vi "VSG_SET-GET_AMPL_1.00.vi"(4 "delay after set (s)":dbl caption="Delay Time (s)", 6 "Get Power Only (T)":bool, 7 "Offset":dbl, 8 "error in":errorcluster {"code" format="%.0x"}, 9 "Set Power (num)":dbl=-25.0, 10 "Set Power(str)":string, 11 "Session In":refnum<visa-resource-name>="GPIB0::18::INSTR") -> (0 "error out":errorcluster {"code" format="%.0x"}, 1 "Get Power":dbl=-25.0, 2 "Get Power (str)":string="-25.000", 3 "Session Out":refnum<visa-resource-name>="GPIB0::18::INSTR")   [LabVIEW 2018]
doc: "Set/Get the ESG RF Amplitude in current units."
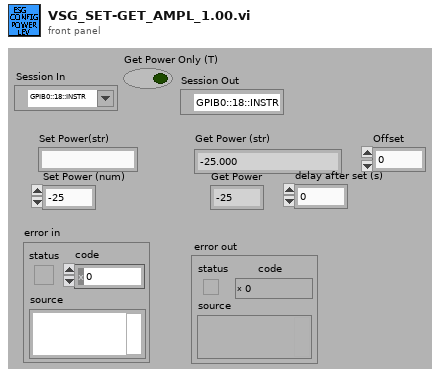
[diagram p1: front panel]
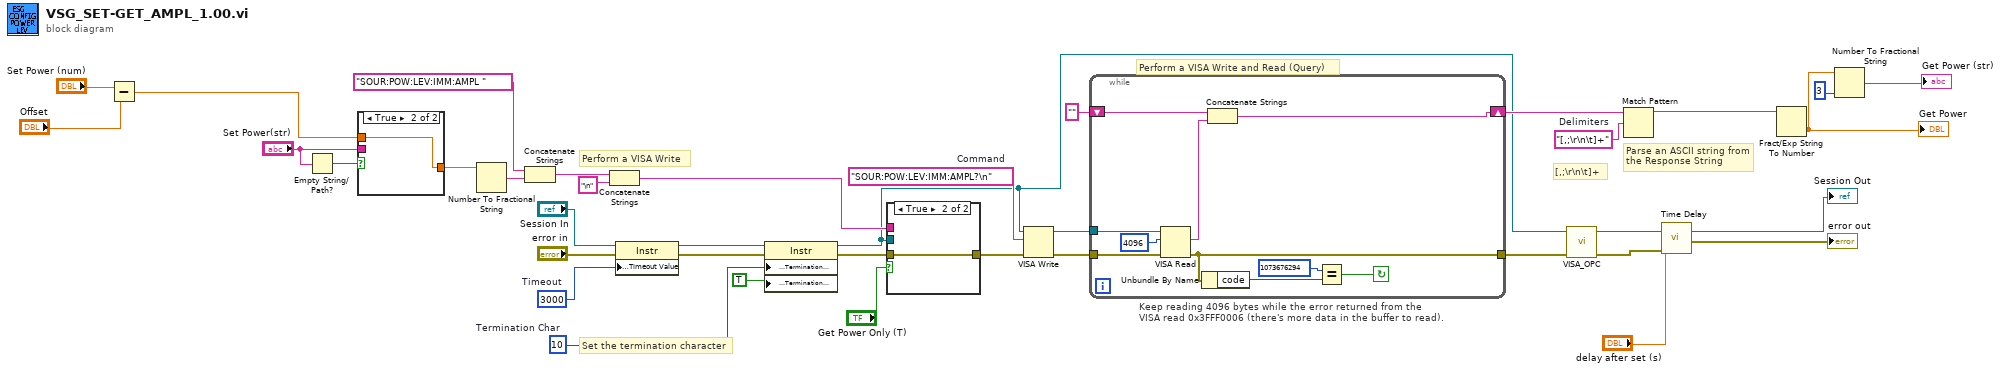
[diagram p0: block diagram]
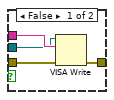
[diagram p2: hidden frame]
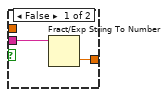
[diagram p3: hidden frame]
diagram:
  w18 = "[,;\r\n\t]+"  # Delimiters
  w19 = "SOUR:POW:LEV:IMM:AMPL?\n"  # Command
  w31 = u8 10  # Termination Char
  w36 = u32 3000  # Timeout
  # "[,;\\r\\n\\t]+"
  # "Parse an ASCII string from the Response String"
  # "Perform a VISA Write and Read (Query)"
  # "Keep reading 4096 bytes while the error returned from the\nVISA read 0x3FFF0006 (there's more data in the buffer to read)."
  # "Perform a VISA Write"
  # "Set the termination character"
  n1 = Subtract(x="Set Power (num)", y="Offset") -> (x-y=w2:dbl)
  n2 = Empty String/Path?(string/path="Set Power(str)") -> (empty?=w14:bool)
  n3 = case shown="True" w14 {
    tunnel: "Set Power(str)" -> [w39 _]
    tunnel: [w38 w40] -> w16
    tunnel: w2 -> [_ w40]
    frame False {
      n4 = Fract/Exp String To Number(string=w39) -> (number=w38:dbl)  [unwired: 3 in, 1 out]
    }
    frame True {
    }
  }
  n5 = Number To Fractional String(number=w16) -> (F-format string=w17:string)  [unwired: 3 in]
  n6 = Concatenate Strings("SOUR:POW:LEV:IMM:AMPL " ("staticText"), w17) -> (w29:string)
  n7 = Concatenate Strings(w29, "\n" ("StaticText")) -> (w26:string)
  n8 = property class="Instr"(reference="Session In", error in="error in", "General Settings:Timeout Value"=w36) -> (reference out=w34:refnum<visa-resource-name>, error out=w33:errorcluster)
  n9 = property class="Instr"(reference=w34, error in=w33, "Message Based Settings:Termination Character"=w31, "Message Based Settings:Termination Character Enable"=TRUE ("enable")) -> (reference out=w11:refnum<visa-resource-name>, error out=w32:errorcluster)
  n10 = case shown="True" "Get Power Only (T)" {
    tunnel: w32 -> [w44 w45]
    tunnel: [w43 w45] -> w27
    tunnel: w26 -> [w42 _]
    tunnel: w11 -> [w41 _]
    frame False {
      n11 = VISA Write(VISA resource name=w41, write buffer=w42, error in (no error)=w44) -> (error out=w43:errorcluster)  [unwired: 2 out]
    }
    frame True {
    }
  }
  n12 = VISA Write(VISA resource name=w11, write buffer=w19, error in (no error)=w27) -> (VISA resource name out=w24:refnum<visa-resource-name>, error out=w22:errorcluster)  [unwired: 1 out]
  n13 = while {
    tunnel: w24 -> [w52]
    shift-right: [w46] -> w23
    shift-left: "" -> [w51]
    tunnel: w22 -> [w49]
    tunnel: [w48] -> w21
    stop <- w47 continue-if-true
    n14 = VISA Read(VISA resource name=w52, byte count=u32 4096 ("byte count (0)"), error in (no error)=w49) -> (read buffer=w50:string, error out=w48:errorcluster)  [unwired: 2 out]
    n15 = Unbundle By Name(w48) -> ("code"=w54:i32)
    n16 = Concatenate Strings(w51, w50) -> (w46:string)
    n17 = Equal?(x=1073676294, y=w54) -> (x = y?=w47:bool)
  }
  n18 = call "VISA_OPC.vi"("error in"=w21, "Session In"=w11) -> ("error out"=w12:errorcluster, "Session Out"=→"Session Out":refnum<visa-resource-name>)  [unwired: 7 in, 1 out]
  n19 = Match Pattern(string=w23, regular expression=w18) -> (before substring=w8:string)  [unwired: 1 in, 3 out]
  n20 = call "Time Delay"("error in (no error)"=w12, "Delay Time (s)"="delay after set (s)") -> ("error out"=→"error out":errorcluster)  [unwired: 9 in]
  n21 = Fract/Exp String To Number(string=w8) -> (number=w7:dbl)  [unwired: 3 in, 1 out]
  "Get Power" <- w7
  n22 = Number To Fractional String(number=w7, precision (6)=i16 3) -> (F-format string=→"Get Power (str)":string)  [unwired: 2 in]
